vi "Test - Draw Textured Triangle.vi"() -> ()   [LabVIEW 2020]
uses:
  Libraries/Utility/Utility.lvlib
  Rectangle Dimensions.ctl
  Raster (FPGA).lvlib
  5ea285c7-be76-47ab-bb95-511c6a9aac96.vi
  d84cddbd-8e40-43c7-a758-6e8d8fd6f2c6.vi
  UV.ctl
  3D/Vector 3D.ctl
  3D/3D (FPGA).lvlib
  3D/Vertex.ctl
  3D/Triangle.ctl
  Texture.ctl
  3D/Material.ctl
panel:
  in  "Triangle":T1={"Vertex 1"={"Position"={"x"=49.0, "y"=26.0, "z"=0.0}, "UV"={"u"=0.739, "v"=0.913}, "Colour"=12517256}, "Vertex 2"={"Position"={"x"=390.0, "y"=98.0, "z"=0.0}, "UV"={"u"=0.317, "v"=0.766}, "Colour"=12517256}, "Vertex 3"={"Position"={"x"=90.0, "y"=303.0, "z"=0.0}, "UV"={"u"=0.814, "v"=0.357}, "Colour"=12517256}, "Alpha"=0.0, "Alpha Blending Enabled"=FALSE, "Colour"=0, "Material"={"Diffuse Colour"=0, "Texture"={"Pixels"=refnum, "Size"={"Width"=0, "Height"=0}}}} {"Vertex 3"."UV"."v" min=0 max=1 step=0.1; "Vertex 3"."UV"."u" min=0 max=1 step=0.1; "Vertex 2"."UV"."v" min=0 max=1 step=0.1; "Vertex 2"."UV"."u" min=0 max=1 step=0.1; "Vertex 1"."UV"."v" min=0 max=1 step=0.1; "Vertex 1"."UV"."u" min=0 max=1 step=0.1}
  out "Time [s]":dbl format="%.3p"
  out "new picture":picture
  # "(0,0)"
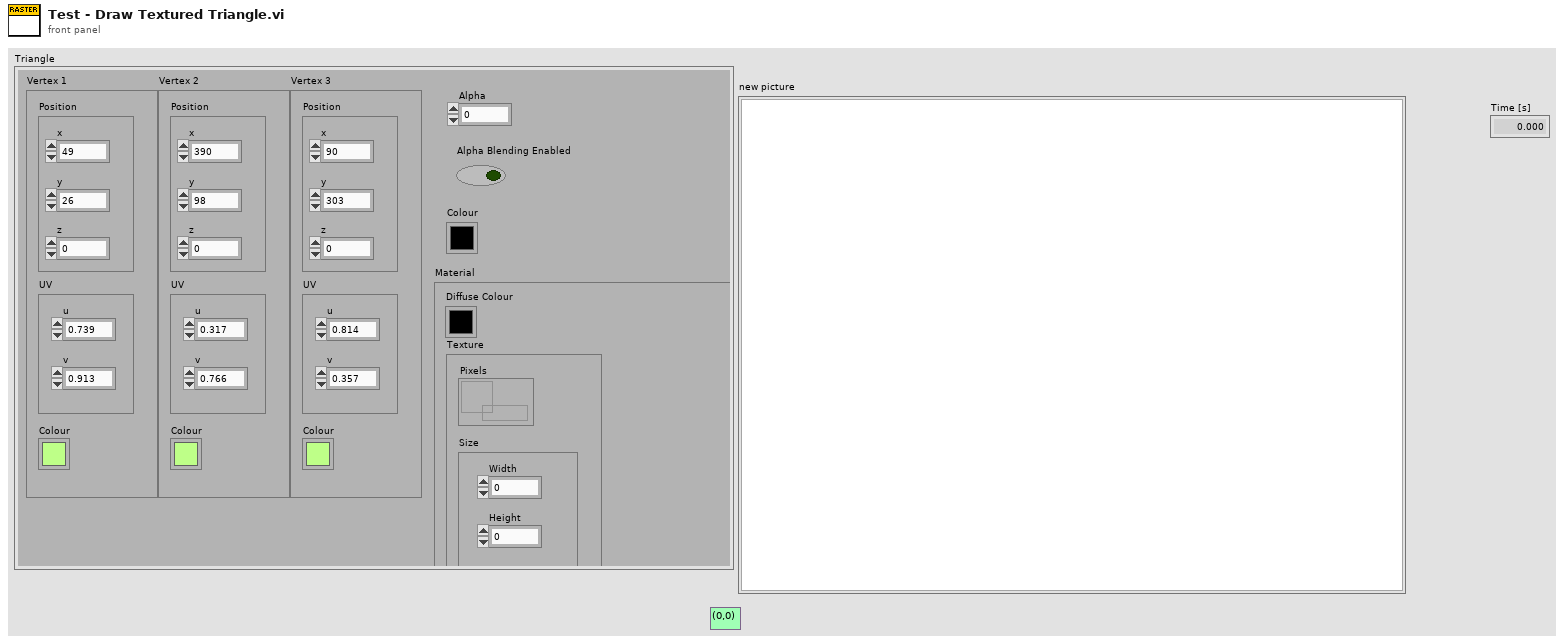
[diagram p1: front panel]
types:
  T1 = typedef "3D (FPGA).lvlib/Triangle.ctl" = cluster{"Vertex 1":T2, "Vertex 2":T2, "Vertex 3":T2, "Alpha":dbl, "Alpha Blending Enabled":bool, "Colour":u32, "Material":T5}
  T2 = typedef "3D (FPGA).lvlib/Vertex.ctl" = cluster{"Position":T3, "UV":T4, "Colour":u32}
  T3 = typedef "3D (FPGA).lvlib/Vector 3D.ctl" = cluster{"x":sgl, "y":sgl, "z":sgl}
  T4 = typedef "Raster (FPGA).lvlib/UV.ctl" = cluster{"u":sgl, "v":sgl}
  T5 = typedef "3D (FPGA).lvlib/Material.ctl" = cluster{"Diffuse Colour":u32, "Texture":T6}
  T6 = typedef "Raster (FPGA).lvlib/Texture.ctl" = cluster{"Pixels":refnum<data-value>, "Size":T7}
  T7 = typedef "Raster (FPGA).lvlib/Rectangle Dimensions.ctl" = cluster{"Width":u32, "Height":u32}
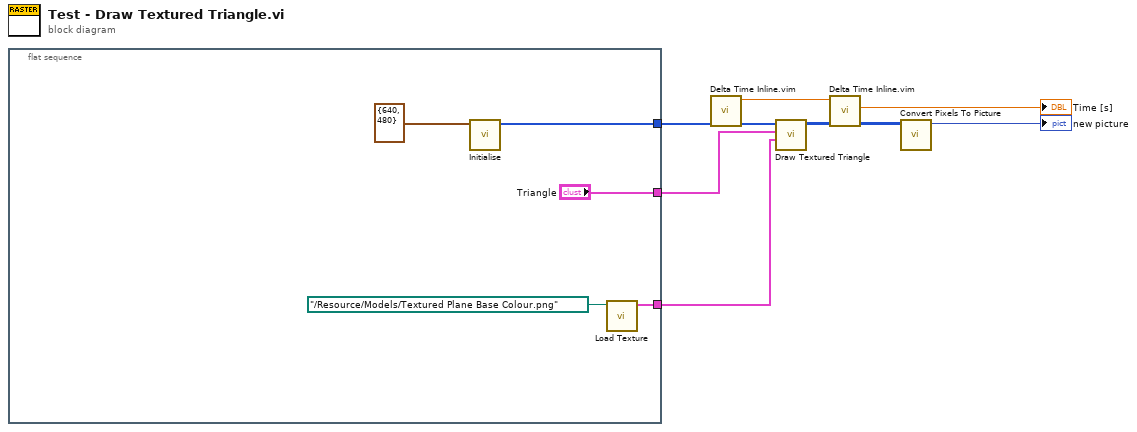
[diagram p0: block diagram]
diagram:
  n1 = flat-sequence {
    tunnel: [w13] -> w8
    tunnel: [w11] -> w2
    tunnel: ["Triangle"] -> w1
    frame #0 {
      n2 = call "Initialise.vi"("Screen Dimensions"=T7 {"Width"=640, "Height"=480}) -> ("Pixel Data out"=w13:u32[])  [unwired: 10 in]
      n3 = call "Load Texture.vi"("Texture Name"=path "../Resource/Models/Textured Plane Base Colour.png" ("name or relative path")) -> ("Texture"=w11:T6)  [unwired: 10 in]
    }
  }
  n4 = call "Delta Time Inline.vim"("value in"=w8) -> ("value out"=w4:u32[], "Relative Seconds out [s]"=w5:dbl)  [unwired: 8 in, 1 out]
  n5 = call "Draw Textured Triangle.vi"("Texture"=w2, "Triangle"=w1, "Pixel Data in"=w4) -> ("Pixel Data out"=w3:u32[][])  [unwired: 8 in]
  n6 = call "Delta Time Inline.vim"("value in"=w3, "Relative Seconds in [s]"=w5) -> ("value out"=w7:u32[][], "Delta Time [s]"=→"Time [s]":dbl)  [unwired: 7 in, 1 out]
  n7 = call "Convert Pixels To Picture.vi"("Pixel Data in"=w7) -> ("2D Picture"=→"new picture":picture)  [unwired: 9 in, 1 out]
